vi "FTW-Endpoint-Multipart-Send.vi"(0 "FTW Endpoint":refnum<class "FTW-Endpoint-TCP.lvclass">, 5 "Message":T1, 7 "Timeout":i32 format="%dmsec", 11 "error in":errorcluster) -> (4 "FTW Endpoint out":refnum<class "FTW-Endpoint-TCP.lvclass">, 6 "Timed out?":bool, 15 "error out":errorcluster)   [LabVIEW 2013, in "FTW-Endpoint-TCP.lvclass"]
uses:
  FTW-Endpoint-TCP.lvclass
  Payload/FTW-MessagePayload.ctl
  FTW-Endpoint-TCP.lvclass/FTW-Endpoint-TCP.ctl
  Error/FTW-ERR-Clear.vi
panel:
  # "Inputs"
  # "Outputs"
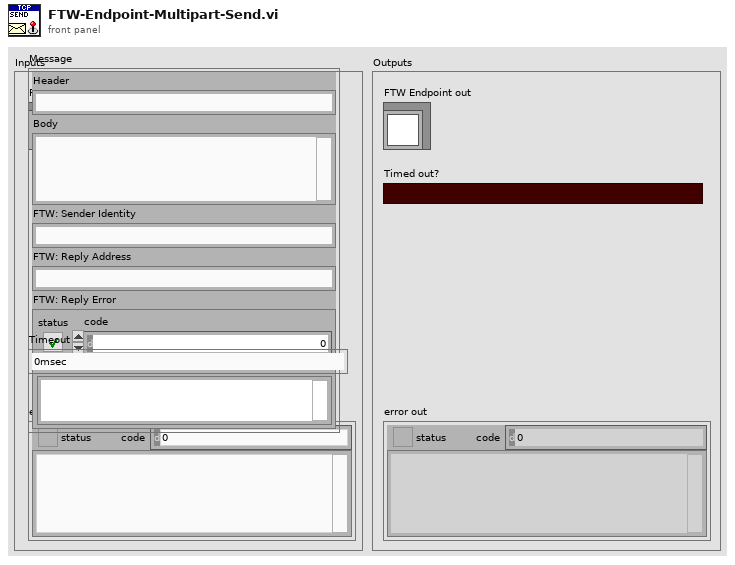
[diagram p1: front panel]
types:
  T1 = typedef "FTW-MessagePayload.ctl" = cluster{"Header":string, "Body":string, "FTW: Sender Identity":string, "FTW: Reply Address":string, "FTW: Reply Error":errorcluster}
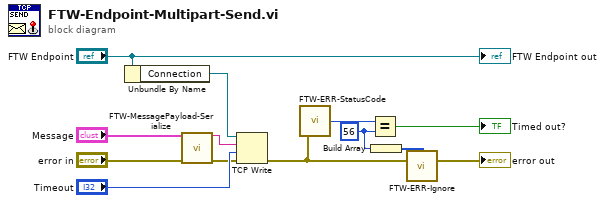
[diagram p0: block diagram]
diagram:
  w3 = 56 ("x")
  n1 = Unbundle By Name("FTW Endpoint") -> ("Connection"=w6:refnum<k5>)
  n2 = call "FTW-MessagePayload-Serialize.vi"("Message In"="Message", "error in"="error in") -> ("Serialized Message"=w5:string, "error out"=w7:errorcluster)  [unwired: 12 in]
  n3 = TCP Write(connection ID=w6, data in=w5, error in (no error)=w7, 9:"Timeout") -> (error out=w1:errorcluster)  [unwired: 2 out]
  n4 = call "FTW-ERR-StatusCode.vi"("error to check"=w1) -> ("Code"=w4:i32)
  n5 = Equal?(x=w4, y=w3) -> (x = y?=→"Timed out?":bool)
  n6 = Build Array(w3) -> (w2:i32[])
  n7 = call "FTW-ERR-Ignore.vi"("Codes to filter"=w2, "error to filter"=w1) -> ("filtered error"=→"error out":errorcluster)  [unwired: 13 in]
  "FTW Endpoint out" <- "FTW Endpoint"
